vi "main 0.2.vi"() -> ()   [LabVIEW 2012]
uses:
  <vilib>/Utility/file.llb/Write To Spreadsheet File (DBL).vi
panel:
  in  "stop":bool
  in  "Path":path
  in  "save":bool
  out "Slide":dbl(slide) scale=0.0..1.0
  in  "count?":bool
  out "img 2":dbl[][](graph)
  in  "snap":bool
  out "Waveform Chart":dbl(graph)
  out "sum":dbl
  in  "dark":bool
  in  "dark imgs":i32
  in  "dark?":bool
  in  "threshold":i32=1
  in  "avg[t] acc[f]":bool
  in  "frames":i32=1
  out "img":dbl[][](graph)
  in  "exp time [s]":dbl=0.01
  in  "binning":dbl=4.0
  in  "close":bool
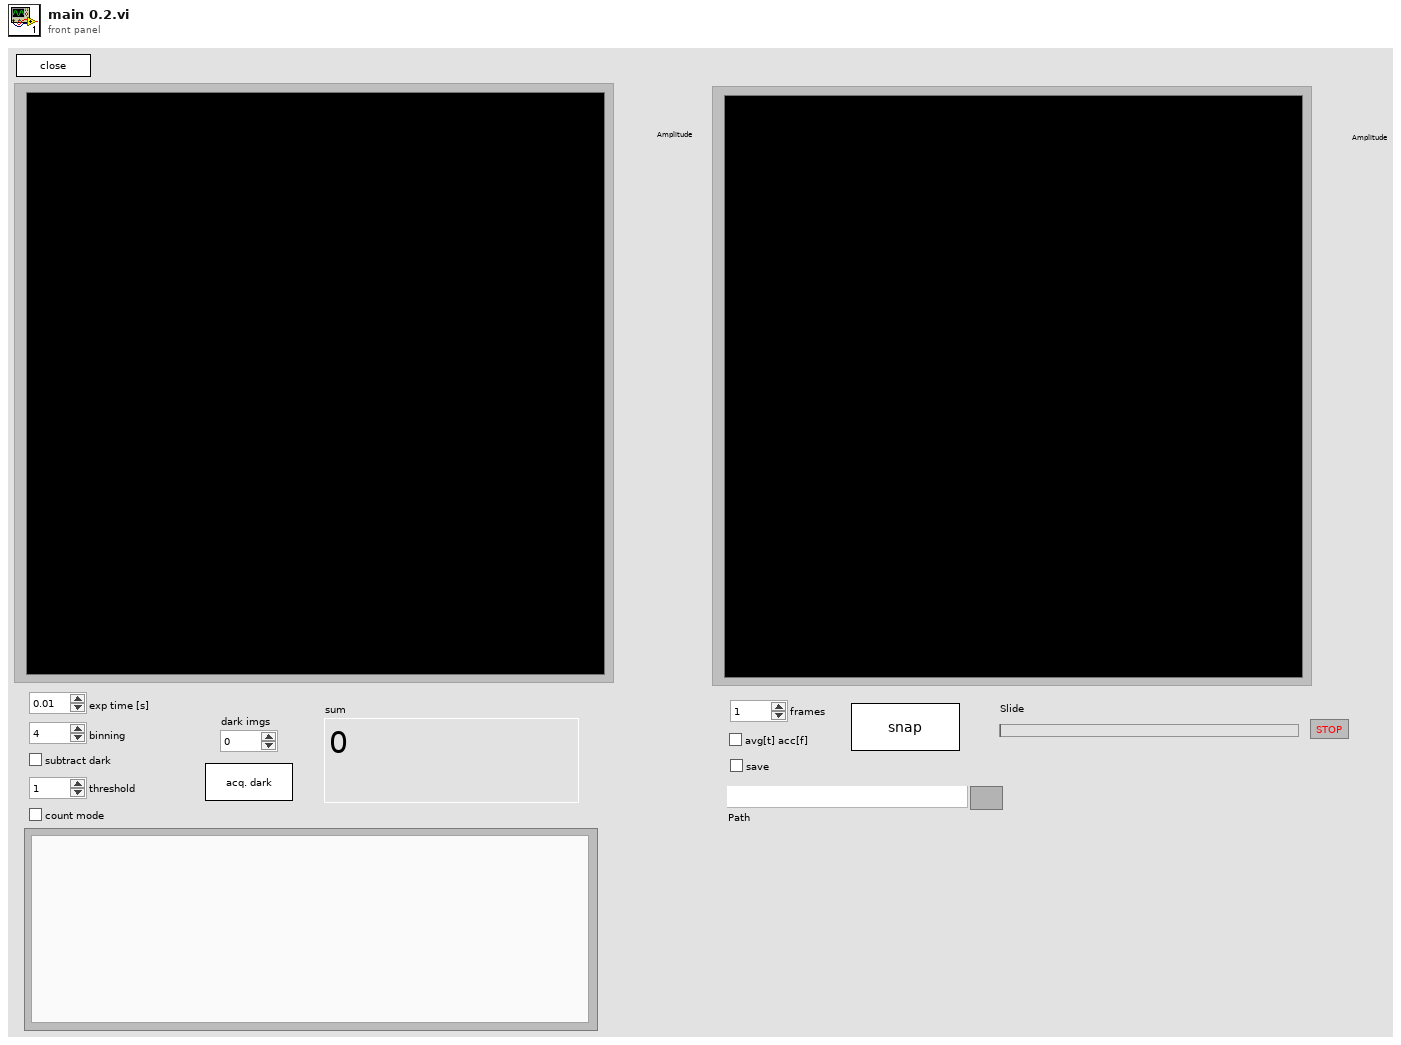
[diagram p1: front panel]
types:
  T1 = cluster{"height":u32, "width":u32, "datatype":u32}
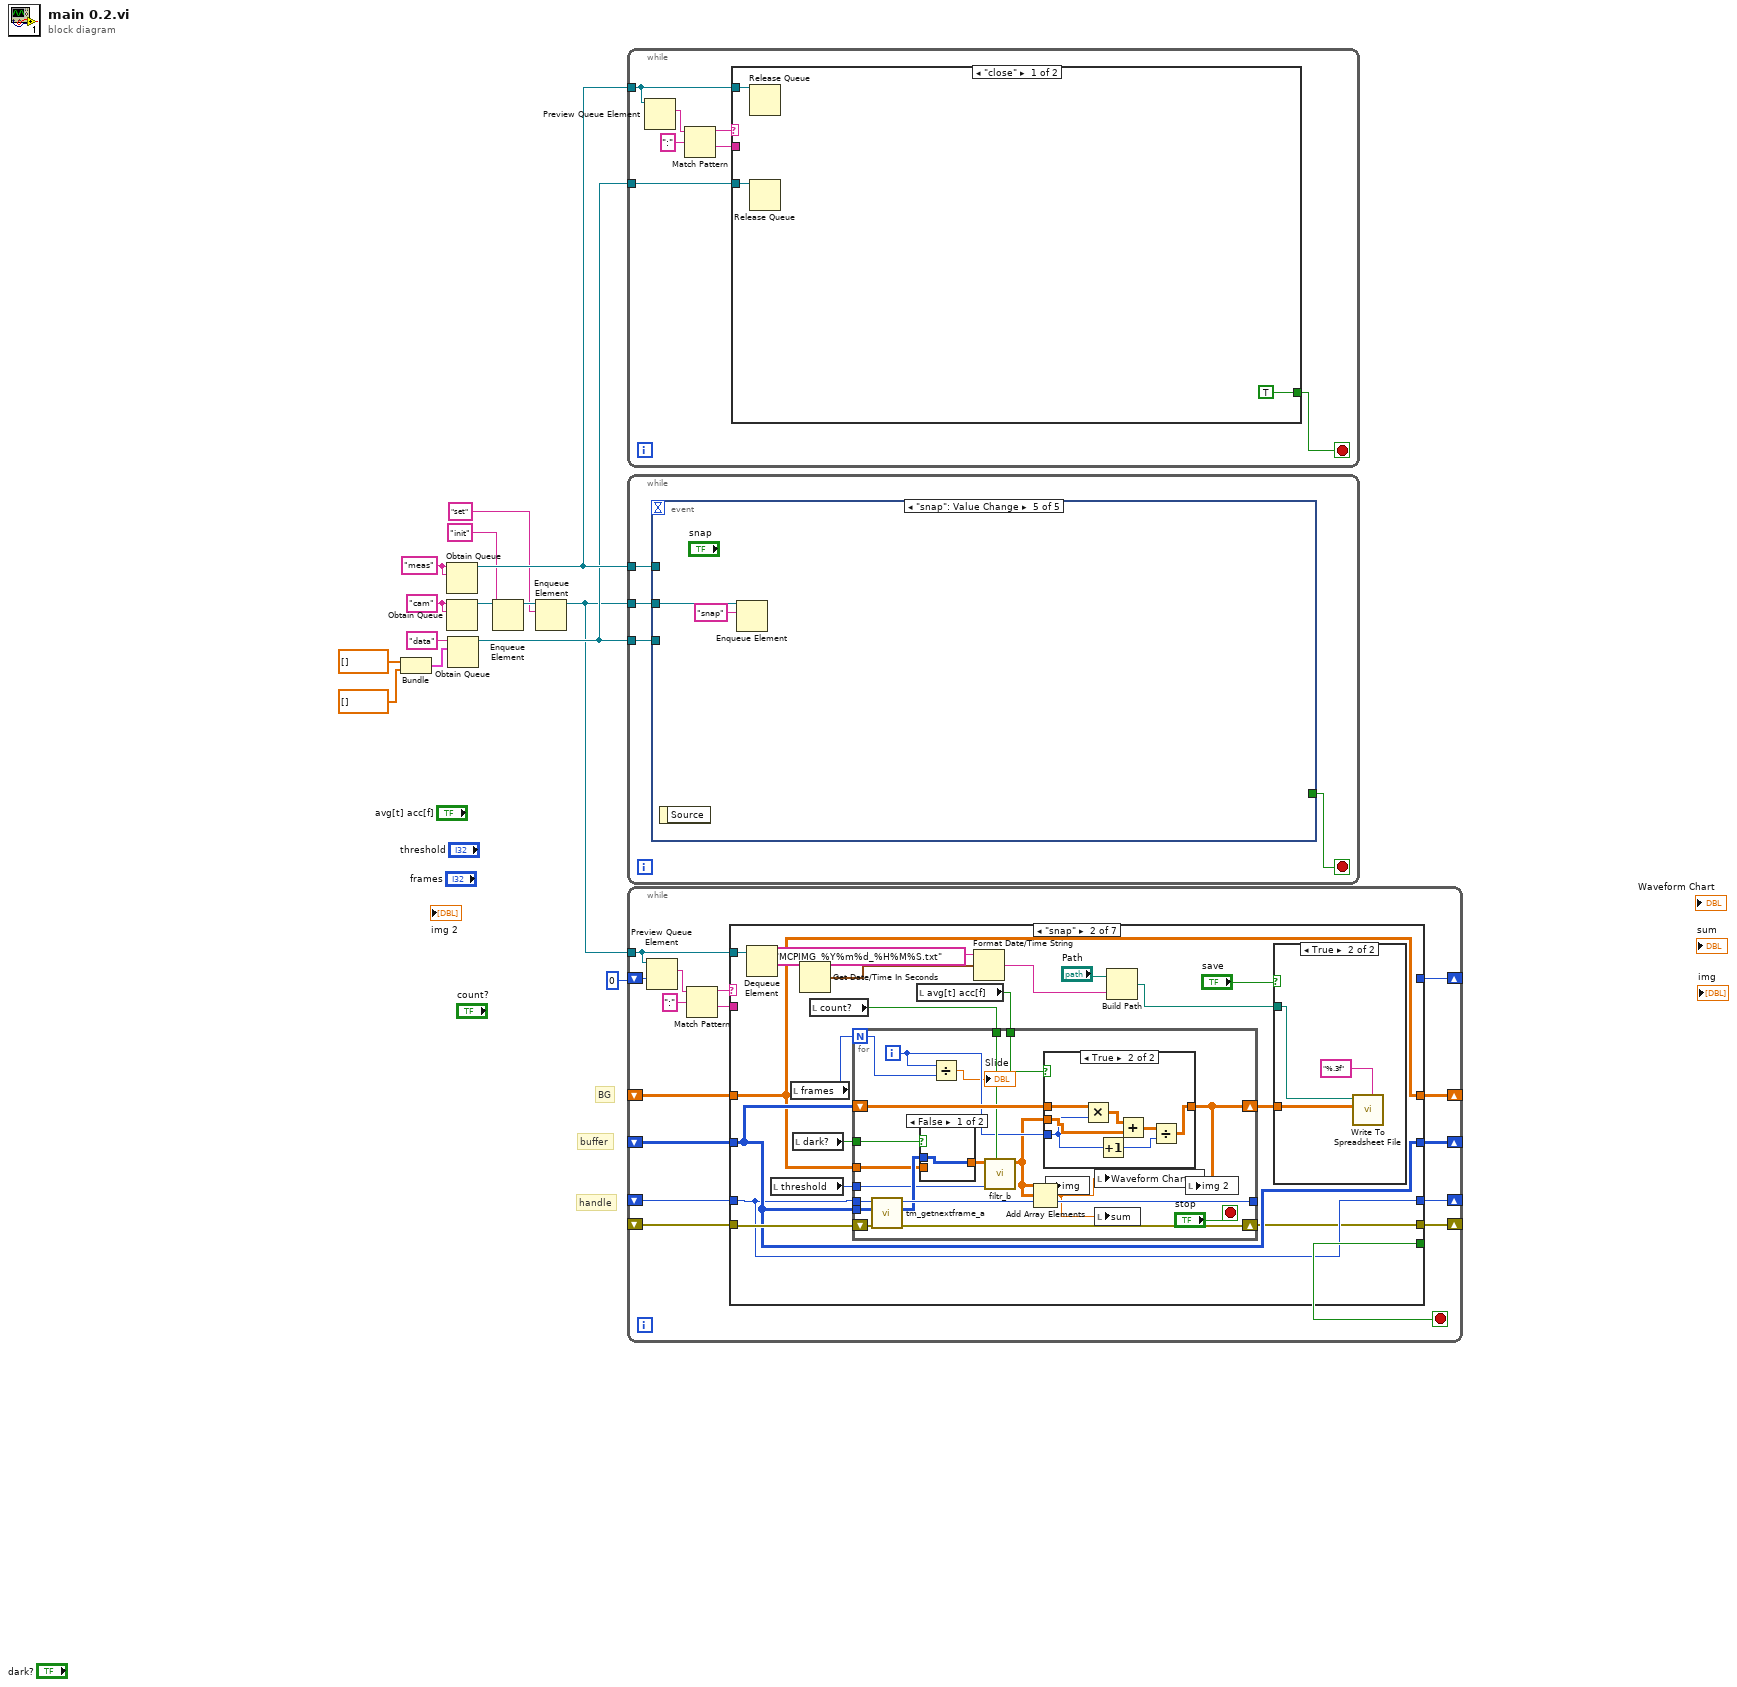
[diagram p0: block diagram]
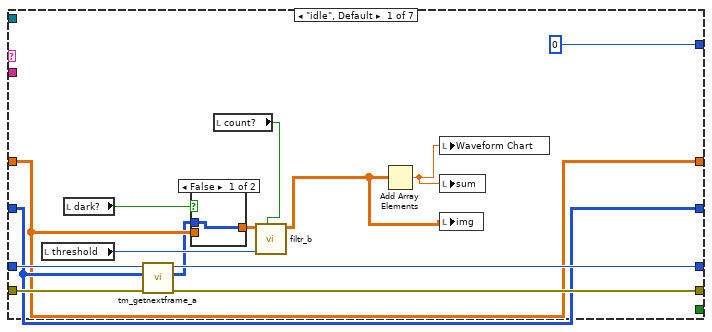
[diagram p3: hidden frame]
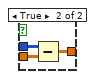
[diagram p4: hidden frame]
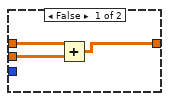
[diagram p6: hidden frame]
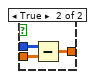
[diagram p7: hidden frame]
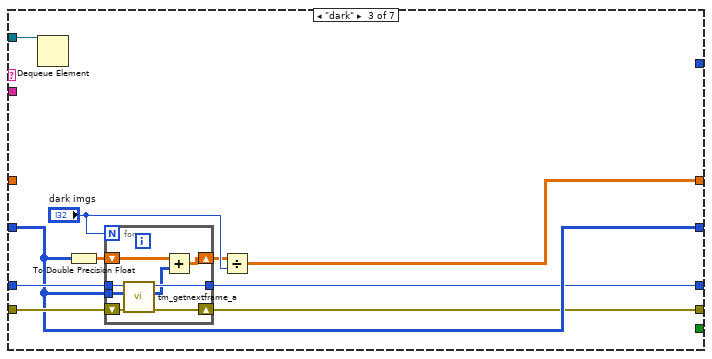
[diagram p8: hidden frame]
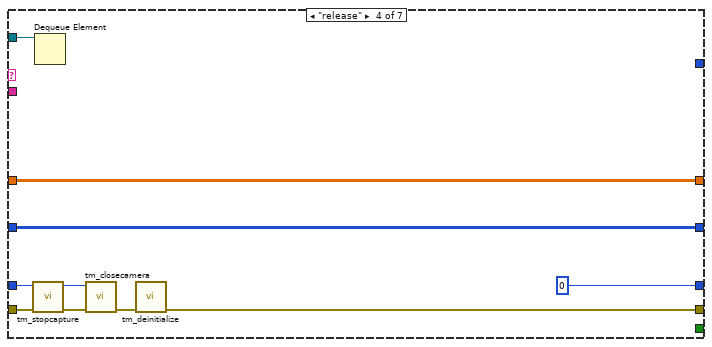
[diagram p9: hidden frame]
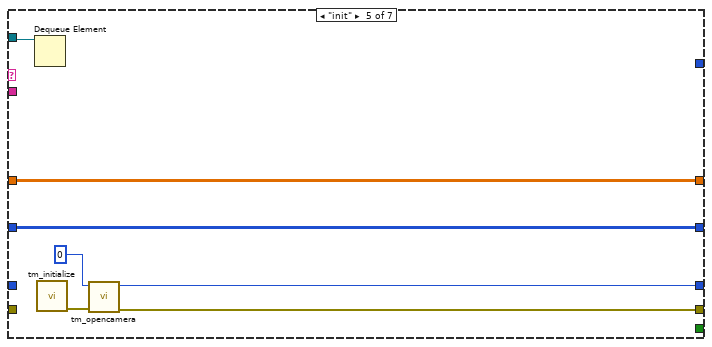
[diagram p10: hidden frame]
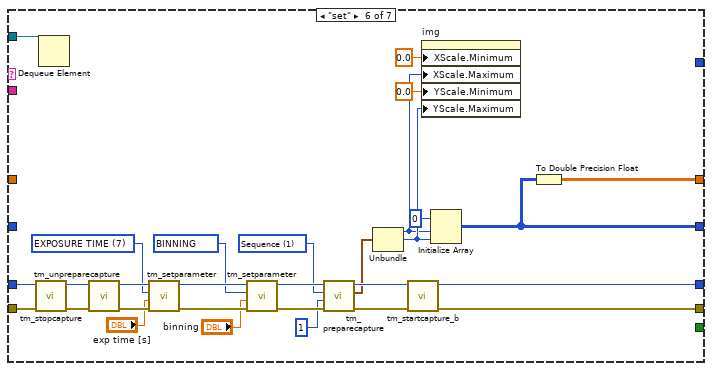
[diagram p11: hidden frame]
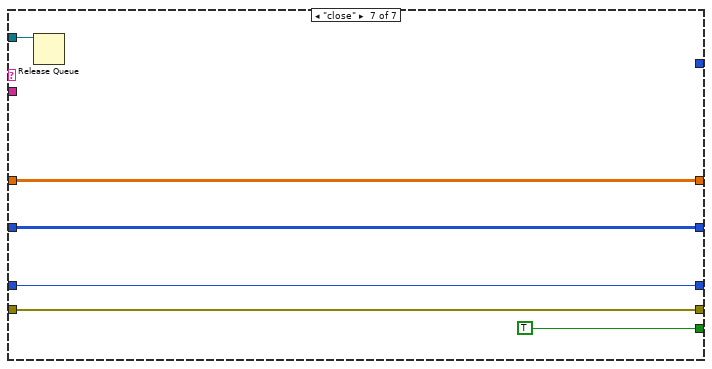
[diagram p12: hidden frame]
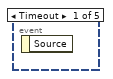
[diagram p13: hidden frame]
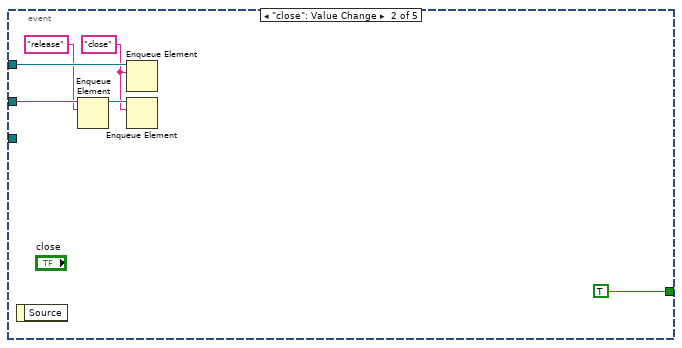
[diagram p14: hidden frame]
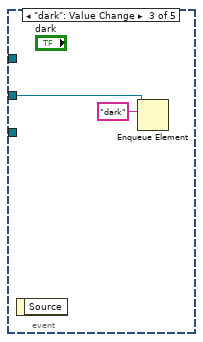
[diagram p15: hidden frame]
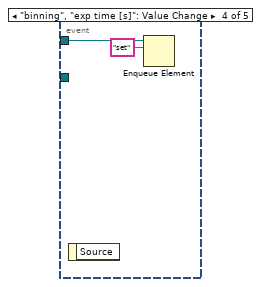
[diagram p16: hidden frame]
diagram:
  w9 = "meas" ("name (unnamed)")
  w12 = "cam" ("name (unnamed)")
  # "BG"
  # "handle"
  # "buffer"
  n1 = Bundle(dbl[] [], dbl[] []) -> (w10:cluster{dbl[], dbl[]})  [unwired: 1 in]
  n2 = Obtain Queue(name (unnamed)=w9, element data type=w9) -> (queue out=w7:refnum<queue>)  [unwired: 3 in, 2 out]
  n3 = Obtain Queue(name (unnamed)=w12, element data type=w12) -> (queue out=w14:refnum<queue>)  [unwired: 3 in, 2 out]
  n4 = Obtain Queue(name (unnamed)="data", element data type=w10) -> (queue out=w6:refnum<queue>)  [unwired: 3 in, 2 out]
  n5 = Enqueue Element(queue=w14, element="init") -> (queue out=w4:refnum<queue>)  [unwired: 2 in, 2 out]
  n6 = Enqueue Element(queue=w4, element="set") -> (queue out=w3:refnum<queue>)  [unwired: 2 in, 2 out]
  n7 = while {
    tunnel: w7 -> [w17]
    tunnel: w6 -> [w16]
    stop <- w15 stop-if-true
    n8 = Preview Queue Element(queue=w17) -> (element=w21:string)  [unwired: 2 in, 3 out]
    n9 = Match Pattern(string=w21, regular expression=":") -> (before substring=w19:string, after substring=w18:string)  [unwired: 1 in, 2 out]
    n10 = case shown="\"close\"" w19 {
      tunnel: w18 -> [_ _]
      tunnel: w17 -> [w23 _]
      tunnel: w16 -> [w24 _]
      tunnel: [TRUE _] -> w15
      frame "close" {
        n11 = Release Queue(queue=w23) -> ()  [unwired: 2 in, 3 out]
        n12 = Release Queue(queue=w24) -> ()  [unwired: 2 in, 3 out]
      }
      frame "idle", Default {
      }
    }
  }
  n13 = while {
    tunnel: w3 -> [w28]
    tunnel: w7 -> [w27]
    tunnel: w6 -> [w26]
    stop <- w25 stop-if-true
    n14 = event shown="[4] \"snap\": Value Change" {
      selector: _ -> [_ _ _ _ _]
      dyn-events: _ -> [_ _ _ _ _]
      timeout: _ -> [_ _ _ _ _]
      tunnel: w28 -> [_ w33 w36 w38 w40]
      tunnel: w27 -> [_ w34 _ _ _]
      tunnel: w26 -> [_ _ _ _ _]
      tunnel: [_ TRUE _ _ _] -> w25
      event Timeout {
        n15 = event-data() -> ()  [unwired: 1 in, 1 out]
      }
      event "close": Value Change {
        w30 = "close" ("element")
        n16 = event-data() -> ()  [unwired: 1 in, 1 out]
        n17 = Enqueue Element(queue=w33, element="release") -> (queue out=w32:refnum<queue>)  [unwired: 2 in, 2 out]
        n18 = Enqueue Element(queue=w34, element=w30) -> ()  [unwired: 2 in, 3 out]
        n19 = Enqueue Element(queue=w32, element=w30) -> ()  [unwired: 2 in, 3 out]
      }
      event "dark": Value Change {
        n20 = event-data() -> ()  [unwired: 1 in, 1 out]
        n21 = Enqueue Element(queue=w36, element="dark") -> ()  [unwired: 2 in, 3 out]
      }
      event "binning", "exp time [s]": Value Change {
        n22 = event-data() -> ()  [unwired: 1 in, 1 out]
        n23 = Enqueue Element(queue=w38, element="set") -> ()  [unwired: 2 in, 3 out]
      }
      event "snap": Value Change {
        n24 = event-data() -> ()  [unwired: 1 in, 1 out]
        n25 = Enqueue Element(queue=w40, element="snap") -> ()  [unwired: 2 in, 3 out]
      }
    }
  }
  n26 = while {
    tunnel: w3 -> [w52]
    shift-right: [w50] -> _
    shift-left: _ -> [w49]
    shift-right: [w48] -> _
    shift-left: _ -> [w47]
    shift-right: [w46] -> _
    shift-left: _ -> [w45]
    shift-right: [w44] -> _
    shift-left: _ -> [w43]
    shift-right: [w41] -> _
    shift-left: 0 -> [w42]
    stop <- w51 stop-if-true
    n27 = Preview Queue Element(queue=w52, timeout in ms (-1)=w42) -> (element=w56:string)  [unwired: 1 in, 3 out]
    n28 = Match Pattern(string=w56, regular expression=":") -> (before substring=w54:string, after substring=w53:string)  [unwired: 1 in, 2 out]
    n29 = case shown="\"snap\"" w54 {
      tunnel: w53 -> [_ _ _ _ _ _ _]
      tunnel: w52 -> [_ w84 w139 w157 w158 w170 w199]
      tunnel: [_ _ _ _ _ _ TRUE] -> w51
      tunnel: [w65 w86 w130 w149 w163 w171 w194] -> w50
      tunnel: w49 -> [w67 w89 w136 w153 _ w193 w194]
      tunnel: [w66 w87 w131 u32 0 ("Handle out") w161 w172 w195] -> w48
      tunnel: w47 -> [w68 w87 w135 w154 _ w191 w195]
      tunnel: [w64 w88 w132 w155 w159 w173 w196] -> w46
      tunnel: w45 -> [w64 w88 w132 w155 w159 _ w196]
      tunnel: [w63 w85 w133 w156 w160 w174 w197] -> w44
      tunnel: w43 -> [w63 w85 _ w156 w160 _ w197]
      tunnel: [0 _ _ _ _ _ _] -> w41
      frame "idle", Default {
        n30 = local read "threshold"() -> (w69:i32)
        n31 = local read "dark?"() -> (w70:bool)
        n32 = call "tm_getnextframe_a.vi"("error in (no error)"=w67, "Buffer"=w64, "Handle in"=w68) -> ("error out"=w65:errorcluster, "Data"=w61:u16[][], "Handle out"=w66:u32)  [unwired: 6 in]
        n33 = case shown="False" w70 {
          tunnel: [w71 w74] -> w60
          tunnel: w61 -> [w71 w73]
          tunnel: w63 -> [_ w72]
          frame False {
          }
          frame True {
            n34 = Subtract(x=w73, y=w72) -> (x-y=w74:dbl[][])
          }
        }
        n35 = local read "count?"() -> (w59:bool)
        n36 = call "filtr_b.vi"("count?"=w59, "threshold"=w69, "input array"=w60) -> ("output array"=w58:dbl[][])  [unwired: 8 in]
        n37 = Add Array Elements(numeric array=w58) -> (sum=w57:dbl)
        n38 = local write "Waveform Chart"(w57) -> ()
        n39 = local write "sum"(w57) -> ()
        n40 = local write "img"(w58) -> ()
      }
      frame "snap" {
        n41 = Dequeue Element(queue=w84) -> ()  [unwired: 2 in, 4 out]
        n42 = local read "threshold"() -> (w91:i32)
        n43 = local read "frames"() -> (w90:i32)
        n44 = local read "dark?"() -> (w92:bool)
        n45 = Get Date/Time In Seconds() -> (seconds since 1Jan1904=w78:timestamp)
        n46 = local read "count?"() -> (w79:bool)
        n47 = local read "avg[t] acc[f]"() -> (w83:bool)
        n48 = for {
          N: w90 -> [w100]
          tunnel: w92 -> [w115]
          tunnel: w88 -> [w113]
          tunnel: w87 -> [w114]
          tunnel: w91 -> [w107]
          tunnel: [w111] -> _
          shift-right: [w110] -> w86
          shift-left: w89 -> [w112]
          tunnel: w85 -> [w106]
          shift-right: [w103] -> w82
          shift-left: w88 -> [w104]
          tunnel: w83 -> [w105]
          tunnel: w79 -> [w102]
          i -> [w101]
          stop <- "stop" stop-if-true
          n49 = call "tm_getnextframe_a.vi"("error in (no error)"=w112, "Buffer"=w113, "Handle in"=w114) -> ("error out"=w110:errorcluster, "Data"=w109:u16[][], "Handle out"=w111:u32)  [unwired: 6 in]
          n50 = case shown="False" w115 {
            tunnel: [w126 w129] -> w108
            tunnel: w109 -> [w126 w128]
            tunnel: w106 -> [_ w127]
            frame False {
            }
            frame True {
              n51 = Subtract(x=w128, y=w127) -> (x-y=w129:dbl[][])
            }
          }
          n52 = Divide(x=w101, y=w100) -> (x/y=→"Slide":dbl)
          n53 = call "filtr_b.vi"("count?"=w102, "threshold"=w107, "input array"=w108) -> ("output array"=w97:dbl[][])  [unwired: 8 in]
          n54 = Add Array Elements(numeric array=w97) -> (sum=w98:dbl)
          n55 = case shown="True" w105 {
            tunnel: w104 -> [w118 w125]
            tunnel: w97 -> [w117 w123]
            tunnel: [w116 w119] -> w103
            tunnel: w101 -> [_ w120]
            frame False {
              n56 = Add(x=w118, y=w117) -> (x+y=w116:dbl[][])
            }
            frame True {
              n57 = Multiply(x=w125, y=w120) -> (x*y=w124:dbl[][])
              n58 = Increment(x=w120) -> (x+1=w121:i32)
              n59 = Add(x=w124, y=w123) -> (x+y=w122:dbl[][])
              n60 = Divide(x=w122, y=w121) -> (x/y=w119:dbl[][])
            }
          }
          n61 = local write "img"(w97) -> ()
          n62 = local write "Waveform Chart"(w98) -> ()
          n63 = local write "sum"(w98) -> ()
          n64 = local write "img 2"(w103) -> ()
        }
        n65 = Format Date/Time String(time format string (%c)="MCPIMG_%Y%m%d_%H%M%S.txt", seconds (now)=w78) -> (date/time string=w76:string)  [unwired: 1 in]
        n66 = Build Path(base path="Path", name or relative path=w76) -> (appended path=w75:path)
        n67 = case shown="True" "save" {
          tunnel: w82 -> [_ w95]
          tunnel: w75 -> [_ w93]
          frame False {
          }
          frame True {
            n68 = call-poly <vilib>:"Write To Spreadsheet File.vi"("format (%.3f)"="%.3f", "2D data"=w95, "file path (dialog if empty)"=w93) -> ()  [unwired: 5 in, 1 out]
          }
        }
      }
      frame "dark" {
        n69 = Dequeue Element(queue=w139) -> ()  [unwired: 2 in, 4 out]
        n70 = To Double Precision Float(number=w132) -> (double precision float=w134:dbl[][])
        n71 = for {
          N: "dark imgs" -> [_]
          tunnel: [w146] -> w131
          shift-right: [w145] -> w130
          shift-left: w136 -> [w147]
          shift-right: [w143] -> w137
          shift-left: w134 -> [w144]
          tunnel: w135 -> [w141]
          tunnel: w132 -> [w140]
          n72 = call "tm_getnextframe_a.vi"("error in (no error)"=w147, "Buffer"=w140, "Handle in"=w141) -> ("error out"=w145:errorcluster, "Data"=w142:u16[][], "Handle out"=w146:u32)  [unwired: 6 in]
          n73 = Add(x=w144, y=w142) -> (x+y=w143:dbl[][])
        }
        n74 = Divide(x=w137, y="dark imgs") -> (x/y=w133:dbl[][])
      }
      frame "release" {
        n75 = call "tm_stopcapture.vi"("error in (no error)"=w153, "Handle in"=w154) -> ("error out"=w151:errorcluster, "Handle out"=w152:u32)  [unwired: 8 in]
        n76 = Dequeue Element(queue=w157) -> ()  [unwired: 2 in, 4 out]
        n77 = call "tm_closecamera.vi"("error in (no error)"=w151, "Handle in"=w152) -> ("error out"=w150:errorcluster)  [unwired: 9 in]
        n78 = call "tm_deinitialize.vi"("error in (no error)"=w150) -> ("error out"=w149:errorcluster)  [unwired: 10 in]
      }
      frame "init" {
        n79 = Dequeue Element(queue=w158) -> ()  [unwired: 2 in, 4 out]
        n80 = call "tm_initialize.vi"() -> ("error out"=w164:errorcluster)  [unwired: 8 in, 3 out]
        n81 = call "tm_opencamera.vi"("error in (no error)"=w164, "Camera Index"=u32 0) -> ("error out"=w163:errorcluster, "Handle out"=w161:u32)  [unwired: 7 in, 1 out]
      }
      frame "set" {
        w179 = 1 items=["Snap", "Sequence"] ("Capture mode")
        w183 = u32 4215968 items=["BINNING"=4215968, "BITS PER CHANNEL"=2, "ACTIVE VIEW INDEX"=3, "CCD MODE"=4, "SENSOR MODE"=5, "READOUT MODE"=6, "EXPOSURE TIME"=7, "CONTRAST GAIN"=8, "CONTRAST OFFSET"=9, "LIGHT MODE"=10, "SENSITIVITY"=11, "WHITE BALANCE"=12, "PHOTON IMAGING MODE"=13, "HIGH DYNAMIC RANGE MODE"=14, "TRIGGER SOURCE"=15, "TRIGGER ACTIVE"=16, "TRIGGER MODE"=17, "TRIGGER POLARITY"=18, "TRIGGER GLOBAL EXPOSURE"=19, "FIRST TRIGGER BEHAVIOR"=20, "TRIGGER TIMES"=21, "OUTPUT TRIGGER POLARITY"=22, "OUTPUT TRIGGER DELAY"=23, "OUTPUT TRIGGER PERIOD"=24, "TEMPERATURE"=25, "TEMPERATURE TARGET"=26, "SENSOR COOLER FAN"=27, "MECHANICAL SHUTTER"=28, "BACK FOCUS POSITION"=29, "FRAMEBUNDLE MODE"=30, "FRAMEBUNDLE NUMBER"=31, "LINEBUNDLE HEIGHT"=32, "TRIGGER CONNECTOR"=33, "IMAGE PIXEL TYPE"=34, "OUTPUT TRIGGER KIND"=35, "READOUT DIRECTION"=36, "CHANNEL SYNC"=37] ("Parameter")
        w187 = u32 7 items=["BINNING"=4215968, "BITS PER CHANNEL"=2, "ACTIVE VIEW INDEX"=3, "CCD MODE"=4, "SENSOR MODE"=5, "READOUT MODE"=6, "EXPOSURE TIME"=7, "CONTRAST GAIN"=8, "CONTRAST OFFSET"=9, "LIGHT MODE"=10, "SENSITIVITY"=11, "WHITE BALANCE"=12, "PHOTON IMAGING MODE"=13, "HIGH DYNAMIC RANGE MODE"=14, "TRIGGER SOURCE"=15, "TRIGGER ACTIVE"=16, "TRIGGER MODE"=17, "TRIGGER POLARITY"=18, "TRIGGER GLOBAL EXPOSURE"=19, "FIRST TRIGGER BEHAVIOR"=20, "TRIGGER TIMES"=21, "OUTPUT TRIGGER POLARITY"=22, "OUTPUT TRIGGER DELAY"=23, "OUTPUT TRIGGER PERIOD"=24, "TEMPERATURE"=25, "TEMPERATURE TARGET"=26, "SENSOR COOLER FAN"=27, "MECHANICAL SHUTTER"=28, "BACK FOCUS POSITION"=29, "FRAMEBUNDLE MODE"=30, "FRAMEBUNDLE NUMBER"=31, "LINEBUNDLE HEIGHT"=32, "TRIGGER CONNECTOR"=33, "IMAGE PIXEL TYPE"=34, "OUTPUT TRIGGER KIND"=35, "READOUT DIRECTION"=36, "CHANNEL SYNC"=37] ("Parameter")
        n82 = call "tm_stopcapture.vi"("error in (no error)"=w193, "Handle in"=w191) -> ("error out"=w192:errorcluster, "Handle out"=w190:u32)  [unwired: 8 in]
        n83 = Dequeue Element(queue=w170) -> ()  [unwired: 2 in, 4 out]
        n84 = call "tm_unpreparecapture.vi"("error in (no error)"=w192, "Handle in"=w190) -> ("error out"=w189:errorcluster, "Handle out"=w188:u32)  [unwired: 8 in]
        n85 = call "tm_setparameter.vi"("error in (no error)"=w189, "Value in"="exp time [s]", "Parameter"=w187, "Handle in"=w188) -> ("error out"=w184:errorcluster, "Handle out"=w185:u32)  [unwired: 6 in]
        n86 = call "tm_setparameter.vi"("error in (no error)"=w184, "Value in"="binning", "Parameter"=w183, "Handle in"=w185) -> ("error out"=w180:errorcluster, "Handle out"=w181:u32)  [unwired: 6 in]
        n87 = call "tm_preparecapture.vi"("error in (no error)"=w180, "Frames"=1, "Capture mode"=w179, "Handle in"=w181) -> ("error out"=w176:errorcluster, "Buffer Info"=w175:T1, "Handle out"=w177:u32)  [unwired: 4 in, 1 out]
        n88 = Unbundle(w175) -> ("height"=w168:u32, "width"=w169:u32)  [unwired: 1 out]
        n89 = call "tm_startcapture_b.vi"("error in (no error)"=w176, "Handle in"=w177) -> ("error out"=w171:errorcluster, "Handle out"=w172:u32)  [unwired: 8 in]
        n90 = property on="img" class="IntGraph (strict)"("XScale.Minimum"=0.0 ("X Scale.Range:Minimum"), "XScale.Maximum"=w168, "YScale.Minimum"=0.0 ("Y Scale.Range:Minimum"), "YScale.Maximum"=w169) -> ()  [unwired: 2 in, 2 out]
        n91 = Initialize Array(u16 0 ("element"), w168, w169) -> (w173:u16[][])
        n92 = To Double Precision Float(number=w173) -> (double precision float=w174:dbl[][])
      }
      frame "close" {
        n93 = Release Queue(queue=w199) -> ()  [unwired: 2 in, 3 out]
      }
    }
  }
